vi "GlobalVariable.vi"() -> ()   [LabVIEW 2014]
panel:
  in  "Fire Override":bool
  in  "WantToSwallow":bool
  in  "Underglow":bool
  in  "Current PSI":dbl
  out "ShooterString":string
  in  "HaloSensitivity":dbl
  in  "BatteryVoltage":dbl
  in  "Ultrasonic":dbl
  in  "Lag Time (ms)":dbl
  in  "GyroAngle":dbl
  in  "WasGoalHot":bool
  in  "AutoShiftAxis":dbl
  in  "AutoShiftHigh":bool
  in  "ArmOverride":bool
  in  "ArmInNXTstate":bool
  in  "IsSpitting":bool
  in  "WantToSpitball":bool
  in  "ArmStateButton":bool
  in  "ShooterCurrentState":T1(ring)
  in  "WantToShoot":bool
  in  "LogShooting":bool
  in  "RollerSpeed":dbl=0.5
  in  "StateDesiredShooter":enum16{"None", "Down", "Up"}(ring)
  in  "Arm State":bool
  in  "Distance":dbl
  out "Shifter H/L":bool
  in  "RightMotorIn":dbl
  in  "LeftMotorIn":dbl
  in  "Velocity":dbl
  in  "Throttle":dbl
  # "Axis 3"
  # "Arm State:\nTrue = Down\nFalse = Up"
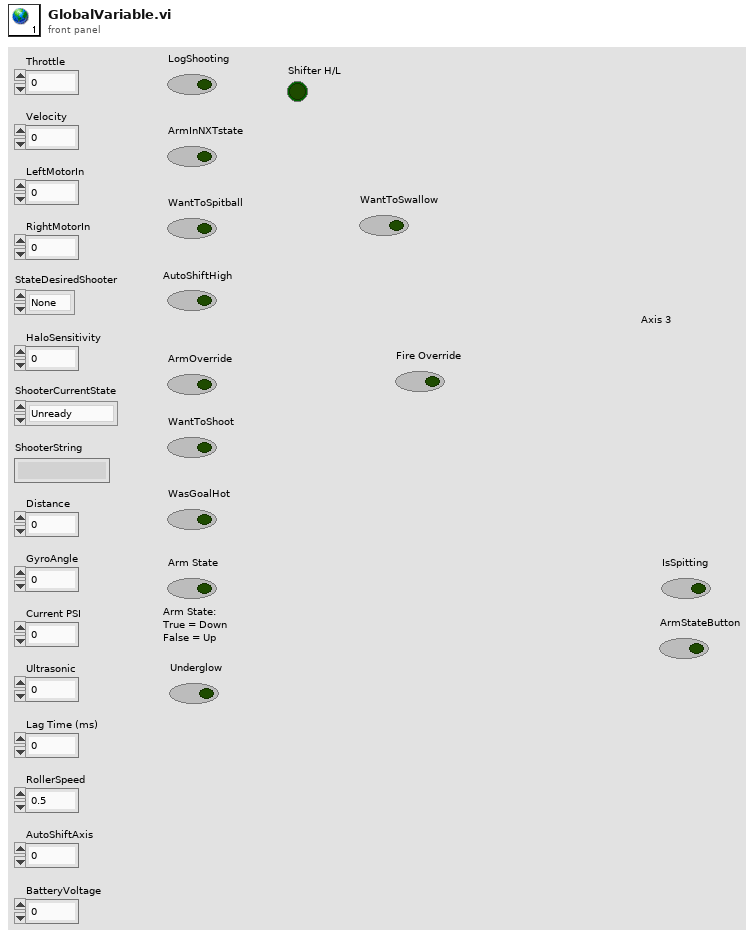
[diagram p1: front panel]
types:
  T1 = enum16{"Unready", "Ready", "Clear", "Fire", "Reload", "Arm In"}
diagram:
